vi "FPGA_SPI_Write_EnableDIO.vi"(8 "error in (no error)":errorcluster, 10 "Enable DIO (F)":bool, 11 "DIO Channel":T1) -> (0 "error out":errorcluster)   [LabVIEW 2017]
uses:
  <vilib>/Rock Robotics/SystemInterfaces/DIO/FPGA_DIOChannel.ctl
  <vilib>/Utility/error.llb/Error Cluster From Error Code.vi
  <vilib>/rvi/errors/niLvFpgaAdjustHostInterfaceError.vi
  <vilib>/rvi/interface/nirviReadWriteControl/nirviReadWriteControl.xnode
  <vilib>/Rock Robotics/SystemInterfaces/System/FPGA_SystemFRC FPGA Ref.ctl
  <vilib>/rvi/interface/Simulation/niFpgaSimulationCallBeginRW.vi
  NiFpgaLv.dll
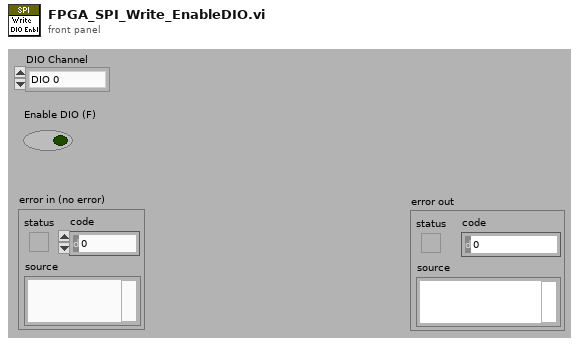
[diagram p1: front panel]
types:
  T1 = typedef "FPGA_DIOChannel.ctl" = enum8{"DIO 0", "DIO 1", "DIO 2", "DIO 3", "DIO 4", "DIO 5", "DIO 6", "DIO 7", "DIO 8", "DIO 9", "DIO MXP 0", "DIO MXP 1", "DIO MXP 2", "DIO MXP 3", "DIO MXP 4", "DIO MXP 5", "DIO MXP 6", "DIO MXP 7", "DIO MXP 8", "DIO MXP 9", "DIO MXP 10", "DIO MXP 11", "DIO MXP 12", "DIO MXP 13", "DIO MXP 14", "DIO MXP 15", "SPI Port CS1", "SPI Port CS2", "SPI Port CS3", "SPI Port MISO", "SPI Port MOSI", "Invalid"}
  T2 = typedef "FPGA_SystemFRC FPGA Ref.ctl" = refnum<k20>
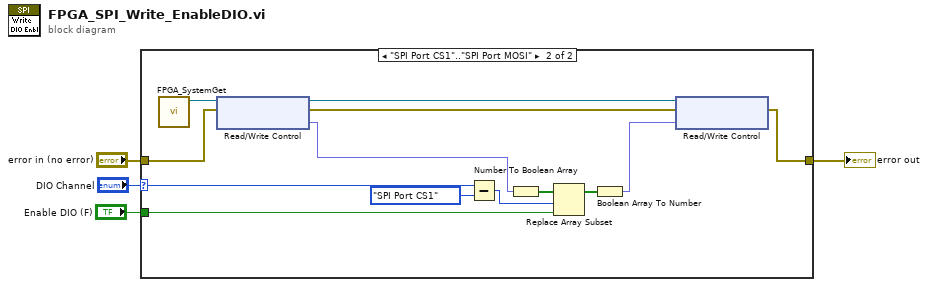
[diagram p0: block diagram]
diagram:
  n1 = case shown="\"SPI Port CS1\"..\"SPI Port MOSI\"" "DIO Channel" {
    selector: "DIO Channel" -> [_ w12]
    tunnel: "error in (no error)" -> [w5 w17]
    tunnel: [w5 w14] -> w3
    tunnel: "Enable DIO (F)" -> [_ w13]
    frame "DIO 0", Default {
      # "change nothing if not a SPI line"
    }
    frame "SPI Port CS1".."SPI Port MOSI" {
      n2 = call <vilib>:"FPGA_SystemGet.vi"() -> ("FRC FPGA Ref"=w18:T2)  [unwired: 11 in]
      n3 = xnode "Read/Write Control"("FPGA VI Reference In"=w18, "error in"=w17) -> ("FPGA VI Reference Out"=w16:T2, "error out"=w15:errorcluster, "SPI.EnableDIO"=w11:fxp<+,5,5>)
      n4 = Subtract(x=w12, y=FPGA_DIOChannel."SPI Port CS1" ("x")) -> (x-y=w7:u8)
      n5 = Number To Boolean Array(number=w11) -> (Boolean array=w9:bool[])
      n6 = Replace Array Subset(array=w9, new element=w13, index=w7) -> (w8:bool[])
      n7 = Boolean Array To Number(Boolean array=w8) -> (number=w10:fxp<+,4,4>)
      n8 = xnode "Read/Write Control"("FPGA VI Reference In"=w16, "error in"=w15, "SPI.EnableDIO"=w10) -> ("error out"=w14:errorcluster)  [unwired: 1 out]
    }
  }
  "error out" <- w3
